vi "SendToPanels.vi"(7 "PanelNumber(-1)":i32=-1, 8 "error in":errorcluster caption="错误输入（无错误）", 9 "Data":variant, 10 "Event":string, 11 "PanelRootNode 输入":refnum<class "PanelRootNode.lvclass"> caption="DNL_LabVIEW Object in") -> (0 "error out":errorcluster caption="错误输出", 3 "PanelRootNode 输出":refnum<class "PanelRootNode.lvclass"> caption="DNL_LabVIEW Object out")   [LabVIEW 2013, in "PanelRootNode.lvclass"]
uses:
  PanelRootNode.lvclass
  share/QueueManager.llb/Insert.vi
  PanelDataNode/PanelDataNode.lvclass
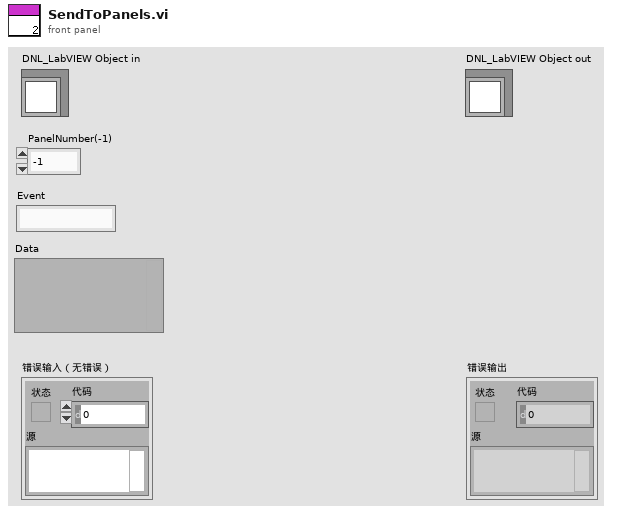
[diagram p1: front panel]
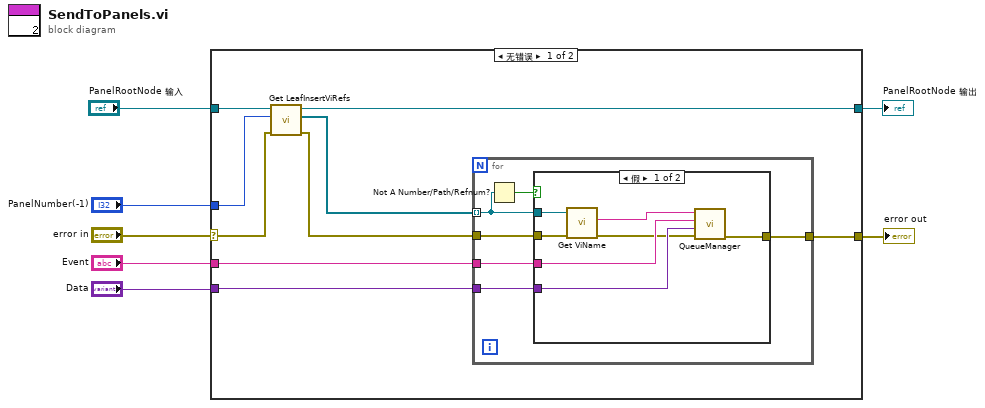
[diagram p0: block diagram]
diagram:
  n1 = case shown="无错误" "error in" {
    selector: "error in" -> [w11 w32]
    tunnel: [w12 w32] -> w6
    tunnel: [w15 w31] -> w4
    tunnel: "PanelRootNode 输入" -> [w16 w31]
    tunnel: "Event" -> [w14 _]
    tunnel: "Data" -> [w13 _]
    tunnel: "PanelNumber(-1)" -> [w9 _]
    frame No Error {
      n2 = call "Get LeafInsertViRefs.vi"("error in (no error)"=w11, "PanelNumber(-1)"=w9, "PanelRootNode 输入"=w16) -> ("error out"=w10:errorcluster, "VI*[]"=w8:refnum<vi>[], "PanelRootNode 输出"=w15:refnum<class "PanelRootNode.lvclass">)  [unwired: 6 in]
      n3 = for {
        tunnel: w8 -> [w22] mode=indexing
        tunnel: w14 -> [w20]
        tunnel: w13 -> [w19]
        tunnel: w10 -> [w18]
        tunnel: [w17] -> w12
        n4 = Not A Number/Path/Refnum?(number/path/refnum=w22) -> (NaN/Path/Refnum?=w21:bool)
        n5 = case shown="假" w21 {
          tunnel: w22 -> [w29 _]
          tunnel: w20 -> [w27 _]
          tunnel: w19 -> [w26 _]
          tunnel: w18 -> [w24 w30]
          tunnel: [w23 w30] -> w17
          frame False {
            n6 = call "Get ViName.vi"("error in"=w24, "VI*"=w29) -> ("error out"=w25:errorcluster, "VI Name"=w28:string)  [unwired: 7 in, 1 out]
            n7 = call-poly "QueueManager.vi"("error in"=w25, "Data"=w26, "Event"=w27, "QueueName"=w28) -> ("error out"=w23:errorcluster)  [unwired: 6 in, 1 out]
          }
          frame True {
          }
        }
      }
    }
    frame Error {
    }
  }
  "error out" <- w6
  "PanelRootNode 输出" <- w4
